vi "Enable Output.vi"(8 "error in (no error)":errorcluster, 10 "Cluster":cluster{"Address":dbl, "Ouput":bool}, 11 "BK-Precision in":refnum<class "BK-Precision.lvclass">) -> (0 "error out":errorcluster, 3 "BK-Precision out":refnum<class "BK-Precision.lvclass">)   [LabVIEW 2021, in "DC PWS.lvlib" / "BK-Precision.lvclass"]
uses:
  BK-Precision.lvclass
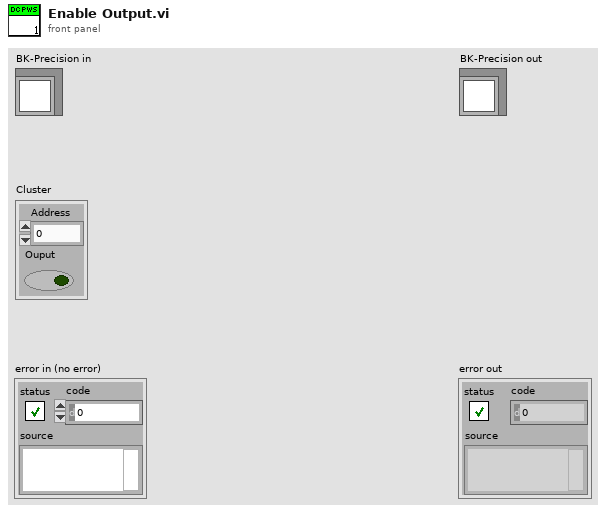
[diagram p1: front panel]
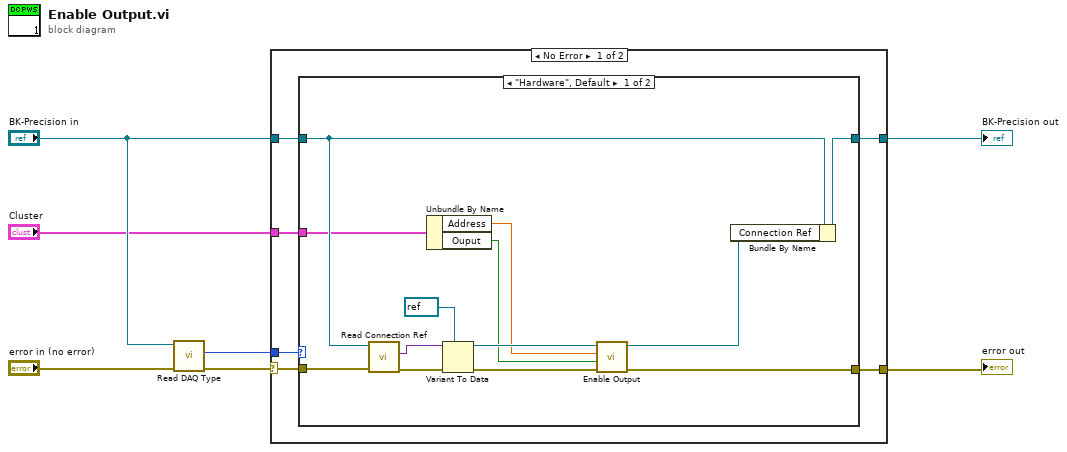
[diagram p0: block diagram]
diagram:
  n1 = call "Read DAQ Type.vi"("error in (no error)"="error in (no error)", "BK-Precision in"="BK-Precision in") -> ("error out"=w6:errorcluster, "Type"=w5:enum16{"Hardware", "Simulation"})  [unwired: 7 in, 1 out]
  n2 = case shown="No Error" w6 {
    selector: w6 -> [w13 w29]
    tunnel: w5 -> [w12 _]
    tunnel: "BK-Precision in" -> [w11 w30]
    tunnel: [w10 w30] -> w3
    tunnel: [w9 w29] -> w2
    tunnel: "Cluster" -> [w8 _]
    frame No Error {
      n3 = case shown="\"Hardware\", Default" w12 {
        tunnel: w13 -> [w26 w27]
        tunnel: w11 -> [w20 w28]
        tunnel: [w18 w28] -> w10
        tunnel: [w19 w27] -> w9
        tunnel: w8 -> [w16 _]
        frame "Hardware", Default {
          n4 = call "Read Connection Ref.vi"("error in (no error)"=w26, "BK-Precision in"=w20) -> ("error out"=w25:errorcluster, "Conn Ref"=w24:variant)  [unwired: 7 in, 1 out]
          n5 = Unbundle By Name(w16) -> ("Address"=w15:dbl, "Ouput"=w14:bool)
          n6 = Variant To Data(error in=w25, type=refnum<visa-resource-name> refnum ("VISA resource name"), Variant=w24) -> (data=w22:refnum<visa-resource-name>, error out=w21:errorcluster)
          n7 = call <instrlib>:"Enable Output.vi"("error in (no error)"=w21, "Enable Output (F: False)"=w14, "Address (0)"=w15, "VISA resource name"=w22) -> ("error out"=w19:errorcluster, "VISA resource name out"=w17:refnum<visa-resource-name>)  [unwired: 6 in]
          n8 = Bundle By Name(cluster=w20, "Connection Ref"=w17) -> (w18:refnum<class "BK-Precision.lvclass">)
        }
        frame "Simulation" {
        }
      }
    }
    frame Error {
    }
  }
  "error out" <- w2
  "BK-Precision out" <- w3
